vi "Unshow Controls as Icons.vi"(8 "error in":errorcluster, 11 "VI Ref":refnum<vi>) -> (0 "error out":errorcluster, 2 "Save?":bool, 3 "VI Ref out":refnum<vi>)   [LabVIEW 2020, in "Code Cleanup.lvlib"]
uses:
  Code Cleanup.lvlib
  <vilib>/Utility/traverseref.llb/VI Scripting - Traverse.lvlib
  <vilib>/Utility/traverseref.llb/TRef TravTarget.ctl
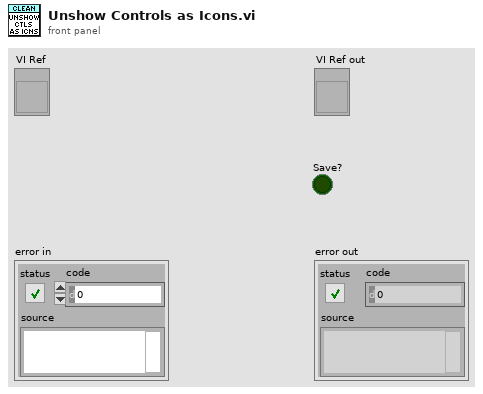
[diagram p1: front panel]
types:
  T1 = typedef "TRef TravTarget.ctl" = enum16{"FP", "BD", "Other"}
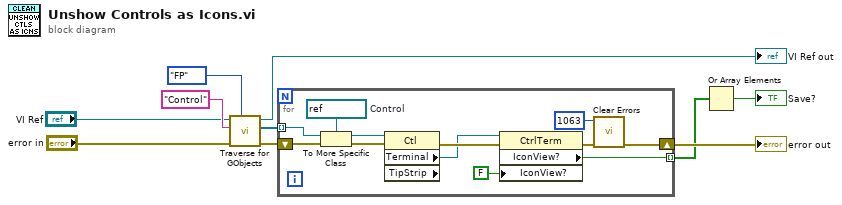
[diagram p0: block diagram]
diagram:
  n1 = call <vilib>:"Traverse for GObjects.vi"("Traverse Target"=TRef_TravTarget."FP", "error in (no error)"="error in", "Class Name"="Control", "VI Refnum"="VI Ref") -> ("error out"=w9:errorcluster, "References"=w6:refnum<vi>[], "dup VI Refnum"=→"VI Ref out":refnum<vi>)  [unwired: 4 in, 1 out]
  n2 = for {
    tunnel: w6 -> [w19] mode=indexing
    shift-right: [w11] -> w5
    shift-left: w9 -> [w22]
    tunnel: [w14] -> w4 mode=indexing
    w18 = refnum<vi> refnum  # Control
    n3 = To More Specific Class(target class=w18, reference=w19, error in=w22) -> (specific class reference=w17:refnum<vi>, error out=w21:errorcluster)
    n4 = property class="Ctl" props=["Terminal", "TipStrip"](reference=w17, error in=w21) -> (error out=w20:errorcluster, "Terminal"=w16:refnum<vi>)  [unwired: 2 out]
    n5 = property class="CtrlTerm"(reference=w16, error in=w20, "IconView?"=FALSE ("Icon View?")) -> (error out=w13:errorcluster, "IconView?"=w14:bool)  [unwired: 1 out]
    n6 = call <vilib>:"Clear Errors.vi"("error in (no error)"=w13, "specific error code to clear (0: all)"=1063) -> ("error out"=w11:errorcluster)  [unwired: 4 in, 1 out]
  }
  "error out" <- w5
  n7 = Or Array Elements(Boolean array=w4) -> (logical OR=→"Save?":bool)
